vi "HexStringtoString.vi"(11 "input String (normal display)":string) -> (3 "output string (hex display)":string)   [LabVIEW 2020, in "IDatabase.lvlib"]
uses:
  IDatabase/IDatabase.lvlib
panel:
  out "output string (normal display)":string
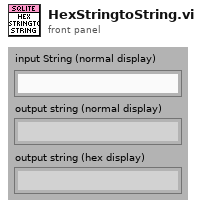
[diagram p1: front panel]
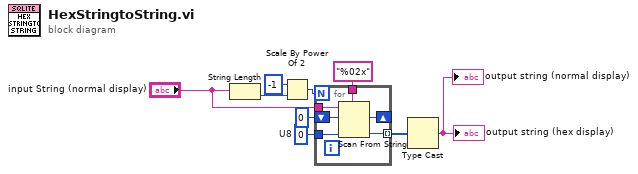
[diagram p0: block diagram]
diagram:
  w8 = u8 0  # U8
  n1 = String Length(string="input String (normal display)") -> (length=w5:i32)
  n2 = Scale By Power Of 2(n=-1, x=w5) -> (x*2^n=w1:i32)
  n3 = for {
    N: w1 -> [_]
    shift-right: [w14] -> _
    shift-left: u32 0 -> [w15]
    tunnel: "input String (normal display)" -> [w13]
    tunnel: w8 -> [w12]
    tunnel: [w11] -> w7 mode=indexing
    tunnel: "%02x" ("format string") -> [w10]
    n4 = Scan From String(format string=w10, input string=w13, initial scan location=w15, default 1=w12) -> (offset past scan=w14:u32, output 1=w11:u8)  [unwired: 1 in, 2 out]
  }
  n5 = Type Cast(x=w7) -> (*(type *) &x=→"output string (hex display)" →"output string (normal display)":string)  [unwired: 1 in]
